vi "Display Results.vi"(8 "error in (no error)":errorcluster, 11 "I-V Result in":refnum<class "I-V Result.lvclass">) -> (0 "error out":errorcluster, 3 "I-V Result out":refnum<class "I-V Result.lvclass">)   [LabVIEW 2015, in "Diode Characterization.lvlib" / "I-V Result.lvclass"]
uses:
  I-V Result.lvclass
  <userlib>/Common Components/Results/Results.lvclass
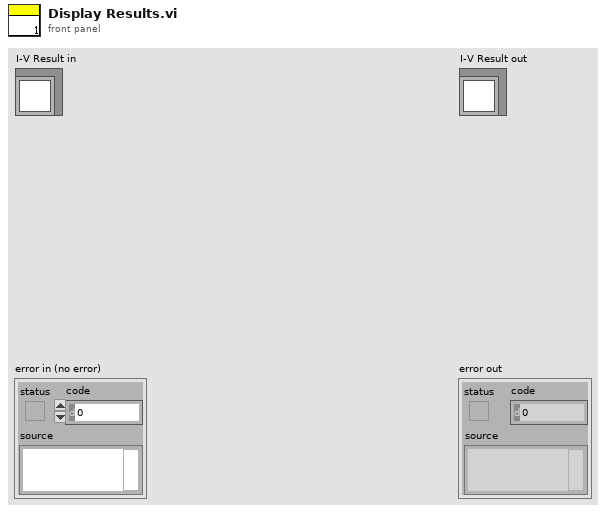
[diagram p1: front panel]
types:
  T1 = typedef "Result Actor.lvlib/Results.lvclass/UI References.ctl" = cluster{"Stop Button":refnum<vi>, "Waveform Graph":refnum<vi>, "Result Name":refnum<vi>, "Pass?":refnum<vi>}
  T2 = typedef "Diode Characterization.lvlib/Diode IV.lvclass/graphdata.ctl" = cluster{"Data":waveform(dbl)[], "AnntList":T3, "CrsrList":T4, "Analysis Data":waveform(dbl)[]}
  T3 = typedef "LVAnnotationListTypeDef.ctl" = cluster{"Name":string, "Color":u32, "Style":u8, "Point Style":u8, "Name Visible":bool, "Allow Drag":bool, "Annotation Mode":u32, "Plot":i32, "Index":i32, "Position":cluster{"X":dbl, "Y":dbl}, "X Scale":u32, "Y Scale":u32, "Show Arrow":bool, "Lock Name":bool, "Plot Area":i32, "Label Offset":cluster{"X":dbl, "Y":dbl}}[]
  T4 = typedef "LVCursorListTypeDef.ctl" = cluster{"Name":string, "Color":u32, "Style":u8, "Point Style":u8, "Name Visible":bool, "Allow Drag":bool, "Cursor Mode":u32, "Plot":i32, "Index":i32, "Position":cluster{"X":dbl, "Y":dbl}, "X Scale":u32, "Y Scale":u32, "Watch Plots":i32[], "Watch All Plots":bool, "Plot Area":i32, "Label Offset":cluster{"X":dbl, "Y":dbl}}[]
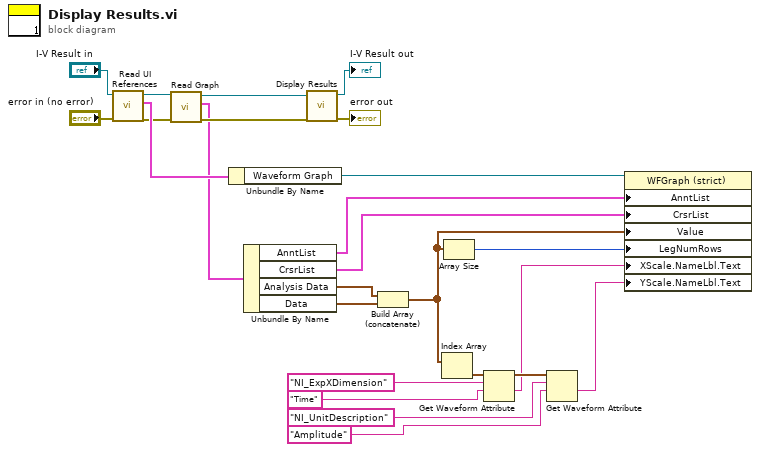
[diagram p0: block diagram]
diagram:
  n1 = call <userlib>:"Read UI References.vi"("error in (no error)"="error in (no error)", "Results in"="I-V Result in") -> ("error out"=w17:errorcluster, "UI References"=w21:T1, "Results out"=w19:refnum<class "I-V Result.lvclass">)  [unwired: 7 in]
  n2 = call "Read Graph.vi"("error in (no error)"=w17, "I-V Result in"=w19) -> ("error out"=w16:errorcluster, "Graph"=w15:T2, "I-V Result out"=w18:refnum<class "I-V Result.lvclass">)  [unwired: 7 in]
  n3 = Unbundle By Name(w21) -> ("Waveform Graph"=w20:refnum<vi>)
  n4 = Unbundle By Name(w15) -> ("AnntList"=w14:T3, "CrsrList"=w13:T4, "Analysis Data"=w12:waveform(dbl)[], "Data"=w11:waveform(dbl)[])
  n5 = call-parent "Display Results.vi"("error in (no error)"=w16, "Results in"=w18) -> ("error out"=→"error out":errorcluster, "Results out"=→"I-V Result out":refnum<class "I-V Result.lvclass">)  [unwired: 8 in]
  n6 = Build Array (concatenate)(w12, w11) -> (w3:waveform(dbl)[])
  n7 = Index Array(array=w3) -> (element=w9:waveform(dbl))  [unwired: 1 in]
  n8 = Array Size(array=w3) -> (size(s)=w10:i32)
  n9 = Get Waveform Attribute(5:"Time", 6:"NI_ExpXDimension", 7:w9) -> (1:w2:string, 3:w7:waveform(dbl))  [unwired: 1 in, 2 out]
  n10 = Get Waveform Attribute(5:"Amplitude", 6:"NI_UnitDescription", 7:w7) -> (1:w1:string)  [unwired: 1 in, 3 out]
  n11 = property class="WFGraph (strict)"(reference=w20, "AnntList"=w14, "CrsrList"=w13, "Value"=w3, "LegNumRows"=w10, "XScale.NameLbl.Text"=w2, "YScale.NameLbl.Text"=w1) -> ()  [unwired: 1 in, 2 out]
